vi "Is State Linked To By.vi"(8 "error in (no error)":errorcluster, 10 "State in":refnum<class "State.lvclass">, 11 "Tosca in":refnum<class "Parameters.lvclass">) -> (0 "error out":errorcluster, 1 "number":i16, 2 "State thru":refnum<class "State.lvclass">, 3 "Tosca thru":refnum<class "Parameters.lvclass">, 4 "linked to?":bool)   [LabVIEW 2015, in "Parameters.lvclass"]
uses:
  Parameters.lvclass
  State/State.lvclass
  Parameters.lvclass/Parameters.ctl
  State/State.lvclass/State.ctl
  State/Read Name.vi
panel:
  out "Array":i32[](array[numeric])
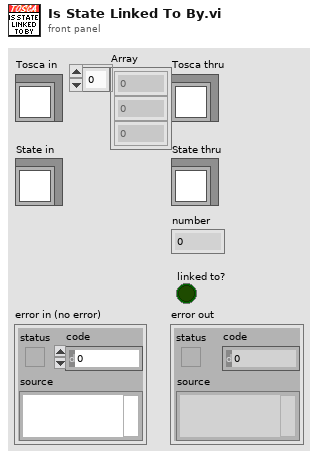
[diagram p1: front panel]
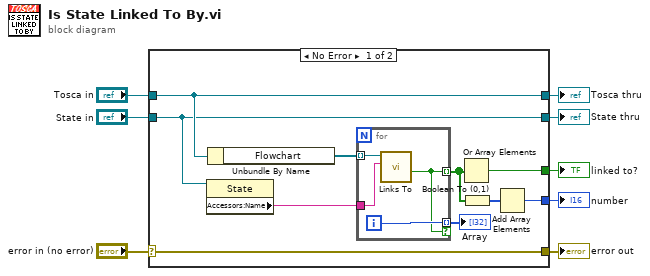
[diagram p0: block diagram]
diagram:
  n1 = case shown="No Error" "error in (no error)" {
    selector: "error in (no error)" -> [w18 w25]
    tunnel: [w18 w25] -> w7
    tunnel: [w17 w24] -> w5
    tunnel: "Tosca in" -> [w17 w24]
    tunnel: "State in" -> [w13 w23]
    tunnel: [w14 _] -> w3
    tunnel: [w13 w23] -> w2
    tunnel: [w10 _] -> w1
    frame No Error {
      n2 = property class="State"(reference=w13) -> ("Accessors:Name"=w15:string)  [unwired: 1 in, 2 out]
      n3 = Unbundle By Name(w17) -> ("Flowchart"=w16:refnum<class "State.lvclass">[])
      n4 = for {
        tunnel: w16 -> [w22] mode=indexing
        tunnel: w15 -> [w21]
        tunnel: [w19] -> w12 mode=indexing
        tunnel: [w20] -> w9 mode=indexing if=w19
        i -> [w20]
        n5 = call "Links To.vi"("State Name"=w21, "State in"=w22) -> ("linked to?"=w19:bool)  [unwired: 7 in, 2 out]
      }
      "Array" <- w9
      n6 = Or Array Elements(Boolean array=w12) -> (logical OR=w14:bool)
      n7 = Boolean To (0,1)(Boolean=w12) -> (0, 1=w11:i16[])
      n8 = Add Array Elements(numeric array=w11) -> (sum=w10:i16)
    }
    frame Error {
    }
  }
  "error out" <- w7
  "Tosca thru" <- w5
  "State thru" <- w2
  "linked to?" <- w3
  "number" <- w1
